vi "OnRestart.vi"(8 "error in (no error)":errorcluster, 11 "Pong in":refnum<class "Pong.lvclass">) -> (0 "error out":errorcluster, 2 "NextGame":refnum<class "Game.lvclass">, 3 "Pong out":refnum<class "Pong.lvclass">)   [LabVIEW 2019, in "RT_Game.lvlib" / "Pong.lvclass"]
uses:
  Pong.lvclass
  C:/Users/FreshBob/Dropbox/VIs/myRIO_GameConsole/RT/RT_Game/Game/Game.lvclass
  Game/Game.lvclass
  Pong.lvclass/Pong.ctl
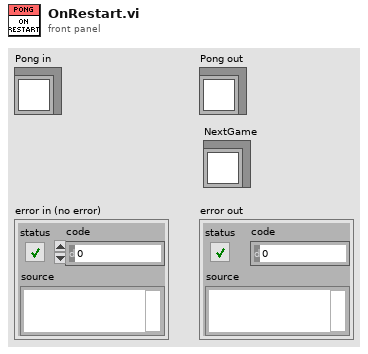
[diagram p1: front panel]
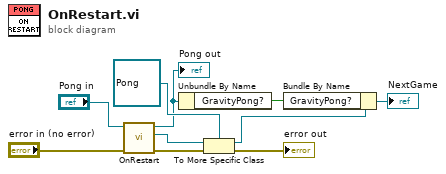
[diagram p0: block diagram]
diagram:
  n1 = call-parent "OnRestart.vi"("error in (no error)"="error in (no error)", "Game in"="Pong in") -> ("error out"=w10:errorcluster, "NextGame"=w6:refnum<class "Game.lvclass">, "Game out"=w2:refnum<class "Pong.lvclass">)  [unwired: 7 in]
  "Pong out" <- w2
  n2 = Unbundle By Name(w2) -> ("GravityPong?"=w1:bool)
  n3 = To More Specific Class(target class=refnum<class "Pong.lvclass"> refnum ("RT_Game.lvlib:Pong.lvclass"), reference=w6, error in=w10) -> (specific class reference=w4:refnum<class "Pong.lvclass">, error out=→"error out":errorcluster)
  n4 = Bundle By Name(cluster=w4, "GravityPong?"=w1) -> (→"NextGame":refnum<class "Pong.lvclass">)
